vi "PeakInterpolate.vi"(10 "Fitting Method":T1 items=["Least Square", "Least Absolute Residual", "Bisquare"], 11 "Data":u16[](array[numeric])) -> (0 "standard deviation":dbl, 2 "Peak (Pseudoindex)":dbl, 3 "Peak (Value)":dbl)   [LabVIEW 2013]
uses:
  <vilib>/Analysis/6fits.llb/Curve Fitting Criteria.ctl
  <vilib>/Analysis/NI_AALPro.lvlib
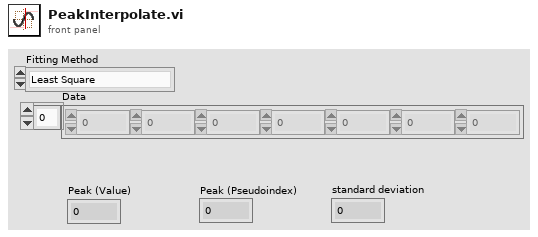
[diagram p1: front panel]
types:
  T1 = typedef "NI_AALPro.lvlib/Curve Fitting Criteria.ctl" = u16
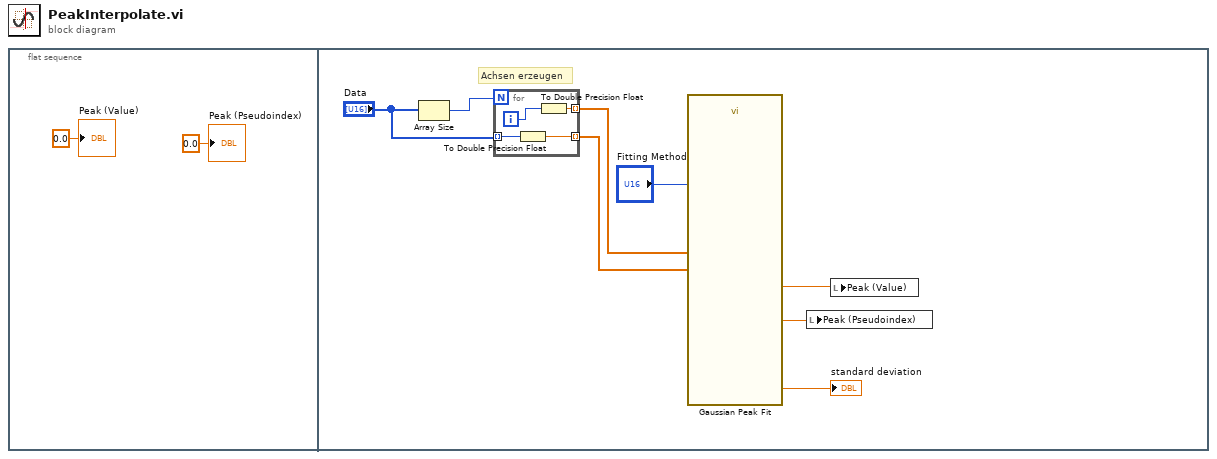
[diagram p0: block diagram]
diagram:
  n1 = flat-sequence {
    frame #0 {
      "Peak (Value)" <- 0.0 ("Maximum (Value)")
      "Peak (Pseudoindex)" <- 0.0 ("Maximum (Index)")
    }
    frame #1 {
      # "Achsen erzeugen"
      n2 = Array Size(array="Data") -> (size(s)=w10:i32)
      n3 = for {
        N: w10 -> [_]
        tunnel: [w13] -> w9 mode=indexing
        tunnel: "Data" -> [w12] mode=indexing
        tunnel: [w11] -> w7 mode=indexing
        i -> [w14]
        n4 = To Double Precision Float(number=w12) -> (double precision float=w11:dbl)
        n5 = To Double Precision Float(number=w14) -> (double precision float=w13:dbl)
      }
      n6 = call <vilib>:"Gaussian Peak Fit.vi"("Y"=w7, "X"=w9, "method"="Fitting Method") -> ("amplitude"=w6:dbl, "center"=w5:dbl, "standard deviation"=→"standard deviation":dbl)  [unwired: 6 in, 4 out]
      n7 = local write "Peak (Pseudoindex)"(w5) -> ()
      n8 = local write "Peak (Value)"(w6) -> ()
    }
  }
